vi "AVI Video-Initialise split file.vi"(8 "error in":errorcluster, 11 "Channel":T1) -> (0 "error out":errorcluster)   [LabVIEW 2013]
uses:
  Typedefs/Channel Selector.ctl
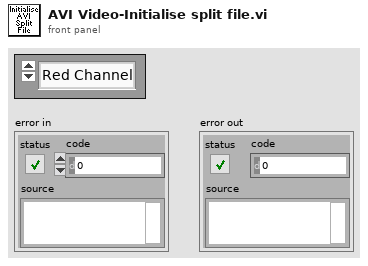
[diagram p1: front panel]
types:
  T1 = typedef "Channel Selector.ctl" = enum16{"Red Channel", "Green Channel", "Blended"}
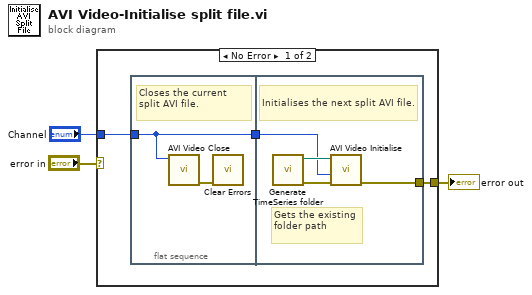
[diagram p0: block diagram]
diagram:
  n1 = case shown="No Error" "error in" {
    selector: "error in" -> [_ w13]
    tunnel: "Channel" -> [w5 _]
    tunnel: [w4 w13] -> w2
    frame No Error {
      n2 = flat-sequence {
        tunnel: w5 -> [w7]
        tunnel: [w7] -> w6
        tunnel: w6 -> [w10]
        tunnel: [w9] -> w4
        frame #0 {
          # "Closes the current split AVI file."
          n3 = call "AVI Video Close.vi"("Channel"=w7) -> ("error out"=w8:errorcluster)  [unwired: 10 in]
          n4 = call <vilib>:"Clear Errors.vi"("error in (no error)"=w8) -> ()  [unwired: 6 in, 1 out]
        }
        frame #1 {
          # "Gets the existing folder path"
          # "Initialises the next split AVI file."
          n5 = call "Generate TimeSeries folder.vi"() -> ("error out"=w12:errorcluster, "Timelapse folder path"=w11:path)  [unwired: 10 in]
          n6 = call "AVI Video Initialise.vi"("error in (no error)"=w12, "Channel"=w10, "Timelapse folder path"=w11) -> ("error out"=w9:errorcluster)  [unwired: 8 in]
        }
      }
    }
    frame Error {
    }
  }
  "error out" <- w2
